vi "WebBroadcast.vi"(6 "MessageQueues":T1, 9 "stds":dbl[](array[numeric]), 10 "Means":dbl[](array[numeric]), 11 "Measure Mode":enum32{"RT Monitor", "IV Monitor"}(ring)) -> ()   [LabVIEW 2024]
uses:
  MessageQueues.ctl
  <vilib>/httpClient/ClientHandle.ctl
  <vilib>/httpClient/POSTBuffer.vi
  <vilib>/httpClient/LabVIEWHTTPClient.lvlib
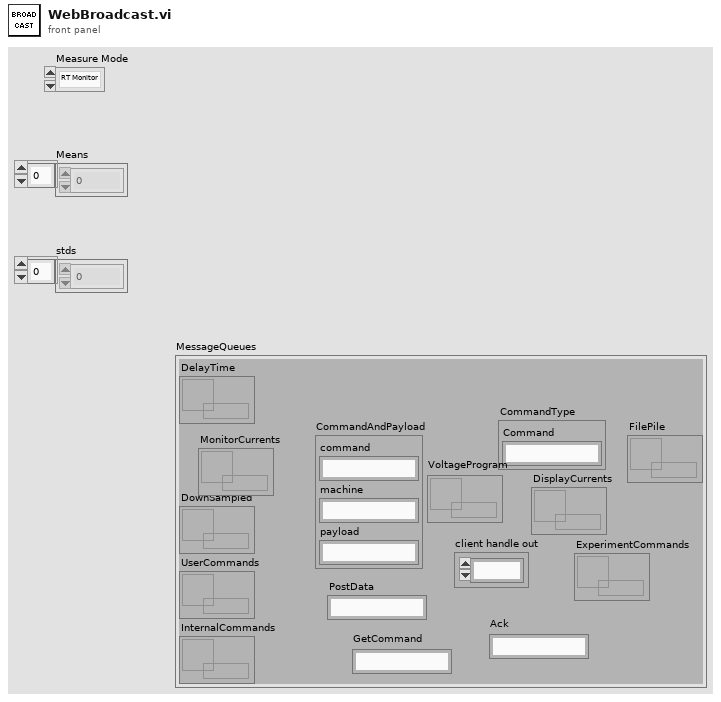
[diagram p1: front panel]
types:
  T1 = typedef "MessageQueues.ctl" = cluster{"DelayTime":refnum<queue>, "DownSampled":refnum<queue>, "UserCommands":refnum<queue>, "InternalCommands":refnum<queue>, "CommandType":cluster{"Command":string}, "CommandAndPayload":cluster{"command":string, "machine":string, "payload":string}, "client handle out":T2, "PostData":string, "GetCommand":string, "Ack":string, "VoltageProgram":refnum<queue>, "ExperimentCommands":refnum<queue>, "DisplayCurrents":refnum<queue>, "MonitorCurrents":refnum<queue>, "FilePile":refnum<queue>}
  T2 = typedef "LabVIEWHTTPClient.lvlib/ClientHandle.ctl" = refnum<k1>
  T3 = cluster{"channelNames":string[], "dt":dbl, "traces":sgl[][], "dataType":string, "means":dbl[], "stds":dbl[]}
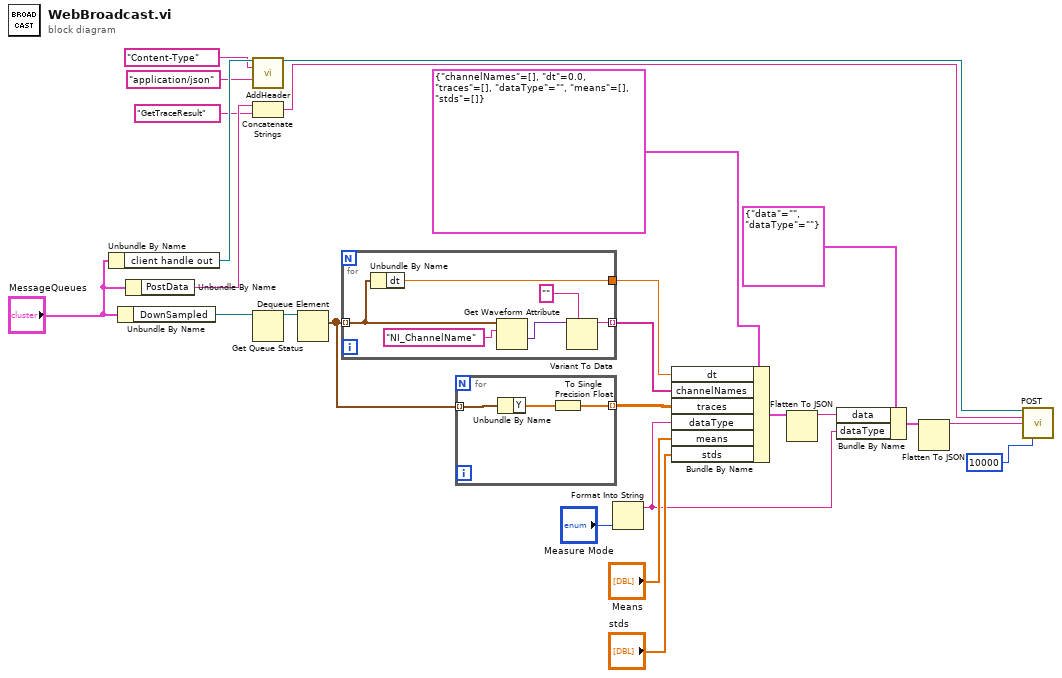
[diagram p0: block diagram]
diagram:
  n1 = Unbundle By Name("MessageQueues") -> ("client handle out"=w23:T2)
  n2 = Unbundle By Name("MessageQueues") -> ("DownSampled"=w22:refnum<queue>)
  n3 = Unbundle By Name("MessageQueues") -> ("PostData"=w24:string)
  n4 = call <vilib>:"AddHeader.vi"("client handle"=w23, "header"="Content-Type", "value"="application/json") -> ("client handle out"=w13:T2)  [unwired: 11 in, 1 out]
  n5 = Concatenate Strings(w24, "GetTraceResult" ("string")) -> (w14:string)
  n6 = Get Queue Status(queue=w22) -> (queue out=w19:refnum<queue>)  [unwired: 2 in, 7 out]
  n7 = Dequeue Element(queue=w19) -> (element=w18:waveform(dbl)[])  [unwired: 2 in, 3 out]
  n8 = for {
    tunnel: w18 -> [w30] mode=indexing
    tunnel: [w31] -> w3
    tunnel: [w27] -> w4 mode=indexing
    n9 = Unbundle By Name(w30) -> ("dt"=w31:dbl)
    n10 = Get Waveform Attribute(6:"NI_ChannelName" ("name"), 7:w30) -> (1:w28:variant)  [unwired: 2 in, 3 out]
    n11 = Variant To Data(type="", Variant=w28) -> (data=w27:string)  [unwired: 1 in, 1 out]
  }
  n12 = for {
    tunnel: w18 -> [w34] mode=indexing
    tunnel: [w32] -> w5 mode=indexing
    n13 = Unbundle By Name(w34) -> ("Y"=w33:dbl[])
    n14 = To Single Precision Float(number=w33) -> (single precision float=w32:sgl[])
  }
  n15 = Format Into String("Measure Mode") -> (resulting string=w17:string)  [unwired: 3 in, 1 out]
  n16 = Bundle By Name(cluster=T3 {"channelNames"=[], "dt"=0.0, "traces"=[], "dataType"="", "means"=[], "stds"=[]}, "dt"=w3, "channelNames"=w4, "traces"=w5, "dataType"=w17, "means"="Means", "stds"="stds") -> (w2:T3)
  n17 = Flatten To JSON(anything=w2) -> (JSON string=w8:string)  [unwired: 2 in, 1 out]
  n18 = Bundle By Name(cluster=cluster{"data":string, "dataType":string} {"data"="", "dataType"=""}, "data"=w8, "dataType"=w17) -> (w9:cluster{"data":string, "dataType":string})
  n19 = Flatten To JSON(anything=w9) -> (JSON string=w10:string)  [unwired: 2 in, 1 out]
  n20 = call-poly <vilib>:"POST.vi"("client handle"=w13, "url"=w14, "buffer"=w10, "timeout (10000)"=10000) -> ()  [unwired: 8 in, 4 out]
